vi "Move_to_pos.vi"(0 "connection ID":refnum<k5>, 1 "Possition selector":T1(radio), 3 "error in":errorcluster) -> (7 "TCP Network Connection out":refnum<k5>, 8 "Driver response":bool, 10 "error out":errorcluster)   [LabVIEW 2019]
panel:
  in  "Cup Position":T2(ring)
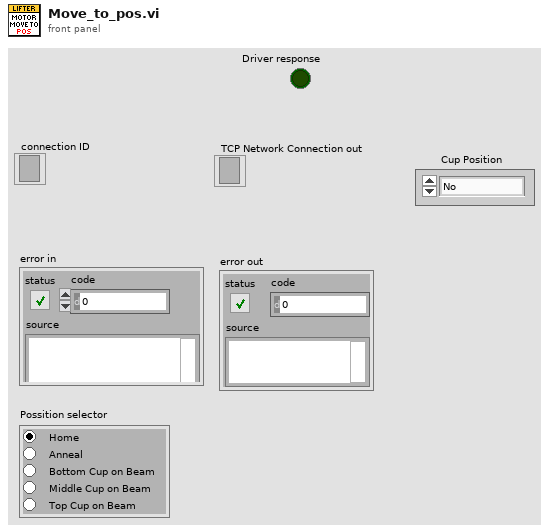
[diagram p1: front panel]
types:
  T1 = enum32{"Home", "Anneal", "Bottom Cup on Beam", "Middle Cup on Beam", "Top Cup on Beam"}
  T2 = enum16{"No", "Home", "Anneal", "Bottom Cup", "Middle Cup", "Top Cup", "Move Up", "Move Down", "Calibrate"}
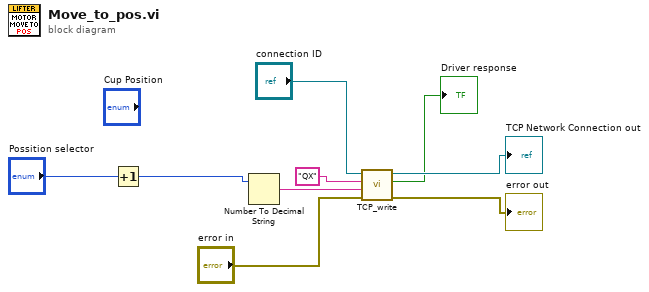
[diagram p0: block diagram]
diagram:
  n1 = Increment(x="Possition selector") -> (x+1=w2:u32)
  n2 = Number To Decimal String(number=w2) -> (decimal integer string=w7:string)  [unwired: 1 in]
  n3 = call "TCP_write.vi"("error in"="error in", "Parameter 2"=w7, "Parameter 1"="QX" ("string"), "connection ID"="connection ID") -> ("error out"=→"error out":errorcluster, "Driver response"=→"Driver response":bool, "TCP Network Connection out"=→"TCP Network Connection out":refnum<k5>)  [unwired: 5 in]
